vi "Readable (No Objects).vi"(8 "error in (no error)":errorcluster, 9 "Channel Units":T2, 10 "Channel Names":T1, 11 "Cluster In":T10={"Channel Names"=[], "Channel Units"=[], "Most Recent Data Points"=[], "History Buffers"=[], "Ring Buffers"=[], "Exp Range Min"=0, "Exp Range Max"=0, "exposure mode"=enum."manual", "operation (meas. mode)"=enum."Measurement mode", "Exposure (ms)"=0, "Quiet Errors?"=FALSE, "Error Status"={"status"=FALSE, "code"=0, "source"=""}}) -> (0 "error out":errorcluster, 3 "Cluster Out":T10={"Channel Names"=[], "Channel Units"=[], "Most Recent Data Points"=[], "History Buffers"=[], "Ring Buffers"=[], "Exp Range Min"=0, "Exp Range Max"=0, "exposure mode"=enum."manual", "operation (meas. mode)"=enum."Measurement mode", "Exposure (ms)"=0, "Quiet Errors?"=FALSE, "Error Status"={"status"=FALSE, "code"=0, "source"=""}})   [LabVIEW 2009]
uses:
  Channel Names.ctl
  Channel Units.ctl
  Data Points.ctl
  Data Point.ctl
  Time.ctl
  X.ctl
  TX Graph.ctl
  Wavelength meter/HighFinesse WS5/Variable Typedefs.llb/Exposure Mode.ctl
  Wavelength meter/HighFinesse WS5/Control typedefs.llb/Measurement Mode.ctl
  Readable.lvclass
  Wavelength meter/HighFinesse WS5/HighFinesse WS5.lvlib
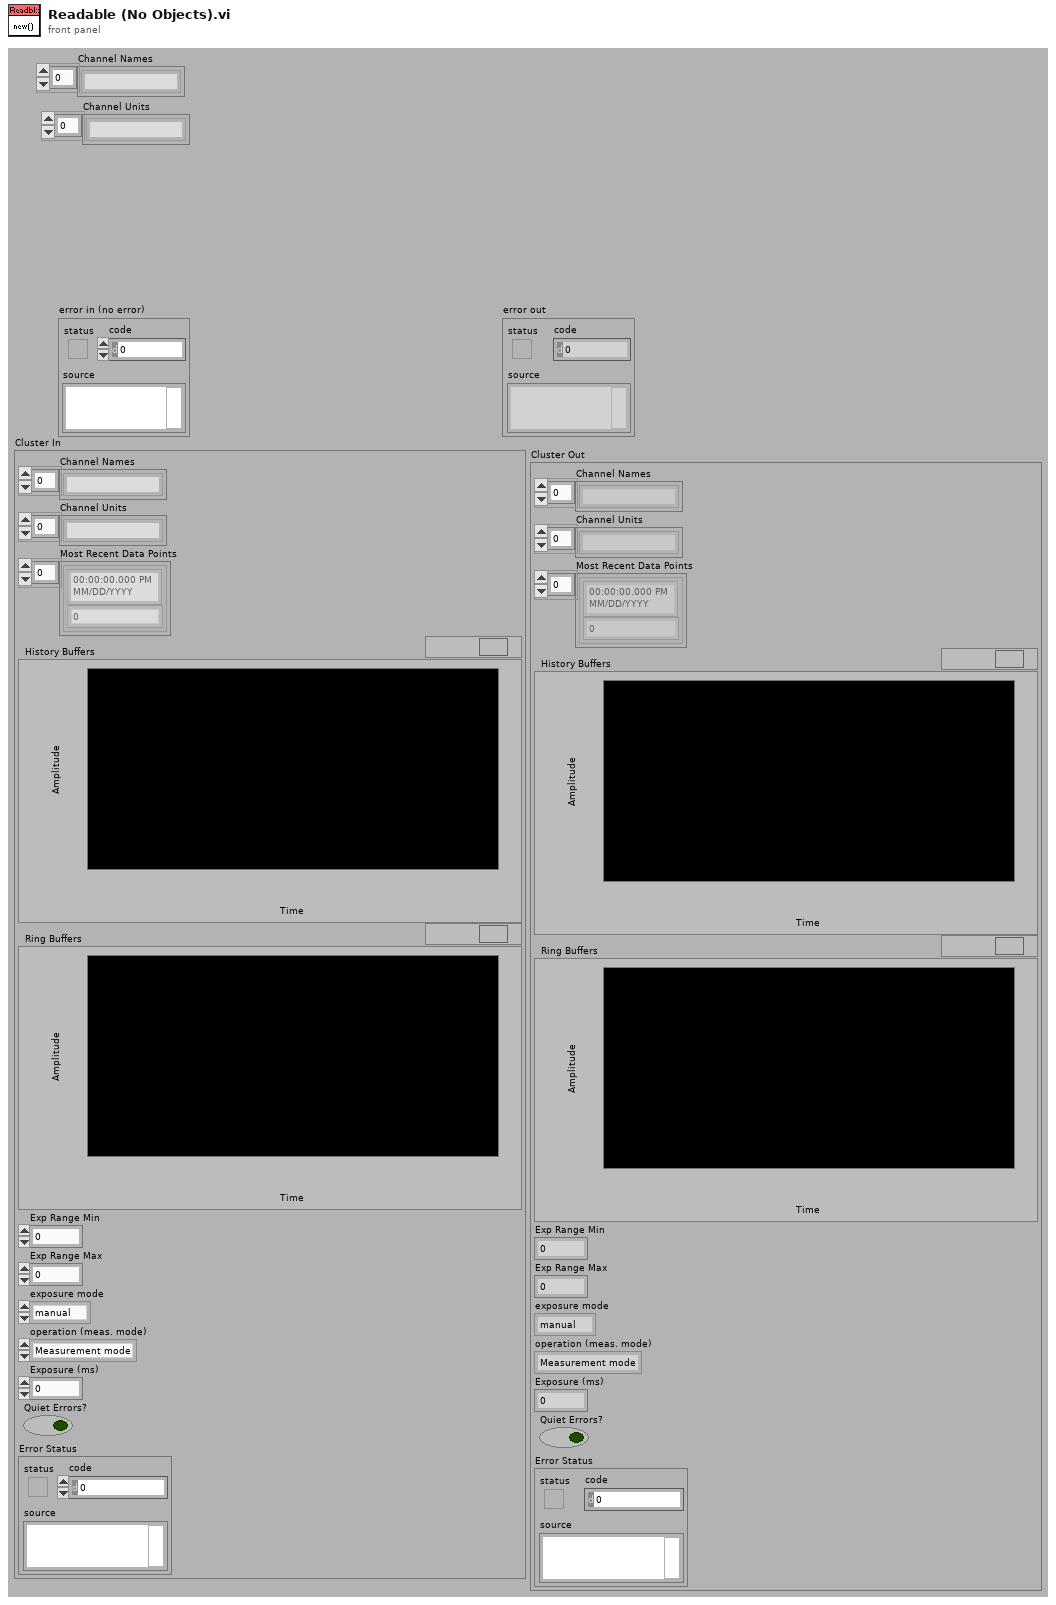
[diagram p1: front panel]
types:
  T1 = typedef "Readable.lvclass/Channel Names.ctl" = string[]
  T2 = typedef "Readable.lvclass/Channel Units.ctl" = string[]
  T3 = typedef "Readable.lvclass/Data Points.ctl" = T4[]
  T4 = typedef "Readable.lvclass/Data Point.ctl" = cluster{"t":T5, "x":T6}
  T5 = typedef "Readable.lvclass/Time.ctl" = timestamp
  T6 = typedef "Readable.lvclass/X.ctl" = dbl
  T7 = typedef "Readable.lvclass/TX Graph.ctl" = cluster{"Data Points":cluster{"t":timestamp, "x":dbl}[]}[]
  T8 = typedef "HighFinesse WS5.lvlib/Exposure Mode.ctl" = enum16{"manual", "automatic"}
  T9 = typedef "HighFinesse WS5.lvlib/Measurement Mode.ctl" = enum16{"Measurement off", "Adjustment mode", "Measurement mode"}
  T10 = cluster{"Channel Names":T1, "Channel Units":T2, "Most Recent Data Points":T3, "History Buffers":T7, "Ring Buffers":T7, "Exp Range Min":u32, "Exp Range Max":u32, "exposure mode":T8, "operation (meas. mode)":T9, "Exposure (ms)":u16, "Quiet Errors?":bool, "Error Status":errorcluster}
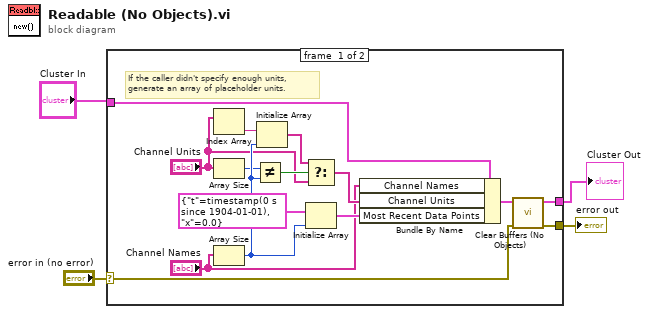
[diagram p0: block diagram]
diagram:
  n1 = case shown="No Error" "error in (no error)" {
    selector: "error in (no error)" -> [w7 w21]
    tunnel: [w6 w21] -> w3
    tunnel: [w8 w20] -> w1
    tunnel: "Cluster In" -> [w19 w20]
    frame #0 {
      # "If the caller didn't specify enough units,\ngenerate an array of placeholder units."
      n2 = Index Array(array="Channel Units") -> (element=w10:string)  [unwired: 1 in]
      n3 = Array Size(array="Channel Units") -> (size(s)=w13:i32)
      n4 = Array Size(array="Channel Names") -> (size(s)=w14:i32)
      n5 = Not Equal?(x=w13, y=w14) -> (x != y?=w12:bool)
      n6 = Initialize Array(w10, w14) -> (w16:string[])
      n7 = Select(t=w16, s=w12, f="Channel Units") -> (s? t:f=w15:T2)
      n8 = Initialize Array(T4 {"t"=timestamp(0 s since 1904-01-01), "x"=0.0} ("Data Point"), w14) -> (w18:T4[])
      n9 = Bundle By Name(cluster=w19, "Channel Names"="Channel Names", "Channel Units"=w15, "Most Recent Data Points"=w18) -> (w5:T10)
      n10 = call "Clear Buffers (No Objects).vi"("error in (no error)"=w7, "Cluster In"=w5) -> ("error out"=w6:errorcluster, "Cluster Out"=w8:T10)  [unwired: 8 in]
    }
    frame #1 {
    }
  }
  "error out" <- w3
  "Cluster Out" <- w1
